vi "Get Manifestation Ancestor Path.vi"(11 "Manifestation Writer in":refnum<class "Manifestation Writer.lvclass">) -> (2 "Manifestation Ancestor Path":path, 3 "Manifestation Writer out":refnum<class "Manifestation Writer.lvclass">)   [LabVIEW 2013, in "Manifestation Writer.lvclass"]
doc: "Copyright (c) 2016 Sze Howe Koh\n\nThis Source Code Form is subject to the terms of the Mozilla Public License, v. 2.0. If a copy of the MPL was not distributed with this file, You can obtain one at http://mozilla.org/MPL/2.0/."
uses:
  Manifestation Writer.lvclass
  Manifestation Writer.lvclass/Manifestation Writer.ctl
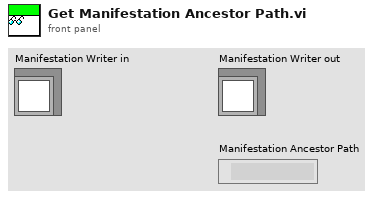
[diagram p1: front panel]
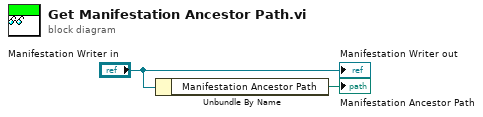
[diagram p0: block diagram]
diagram:
  n1 = Unbundle By Name("Manifestation Writer in") -> ("Manifestation Ancestor Path"=→"Manifestation Ancestor Path":path)
  "Manifestation Writer out" <- "Manifestation Writer in"
